vi "Extract RSSI Measurement from String.vi"(11 "Normal Event Log String":string="LogNum=1\r\nCount=7\r\nSerial=0\r\n\r\nTimestamp=4472778\r\nEvent=2308\r\nDescription= E_LOG_MICS_RSSI\r\nEventData[0]=1E\r\nEventData[1]=00\r\nEventData[2]=00\r\nEventData[3]=00\r\n\r\nTimestamp=4472802\r\nEvent=2308\r\nDescription= E_LOG_MICS_RSSI\r\nEventData[0]=0B\r\nEventData[1]=00\r\nEventData[2]=00\r\nEventData[3]=00\r\n\r\nTimestamp=4472828\r\nEvent=2308\r\nDescription= E_LOG_MICS_RSSI\r\nEventData[0]=00\r\nEventData[1]=00\r\nEventData[2]=00\r\nEventData[3]=00\r\n\r\nTimestamp=4472854\r\nEvent=2308\r\nDescription= E_LOG_MICS_RSSI\r\nEventData[0]=00\r\nEventData[1]=00\r\nEventData[2]=00\r\nEventData[3]=00\r\n\r\nTimestamp=4475025\r\nEvent=2121\r\nDescription= Event log was read\r\nEventData[0]=00\r\nEventData[1]=00\r\nEventData[2]=00\r\nEventData[3]=00\r\n\r\nTimestamp=9513895\r\nEvent=2121\r\nDescription= Event log was read\r\nEventData[0]=00\r\nEventData[1]=00\r\nEventData[2]=00\r\nEventData[3]=00\r\n\r\nTimestamp=9578215\r\nEvent=2121\r\nDescription= Event log was read\r\nEventData[0]=00\r\nEventData[1]=00\r\nEventData[2]=00\r\nEventData[3]=00") -> (2 "RSSI Values":u32[](array[numeric]), 3 "RSSI Values (String, HEX)":string[](array[string]))   [LabVIEW 2010]
doc: "This function converts a string containg the IPG VBAT ADC count into volts.\n\nThe IPG VBAT ADC is 12-bit unsigned, full scale is 5.00 volts.\nThe ADC scale factor is 0.001221001 per ADC bit. (4095 * 0.001221001 = 5.0000 volts)"
panel:
  out "tokens":string[](array[string])
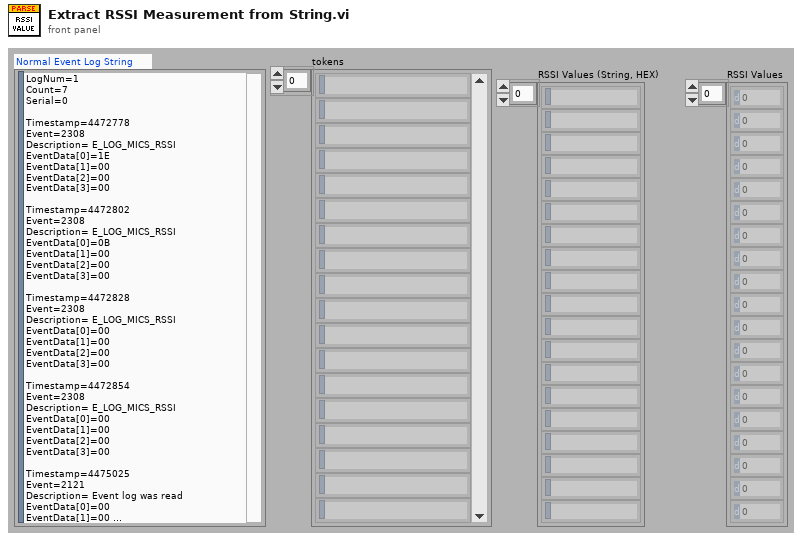
[diagram p1: front panel]
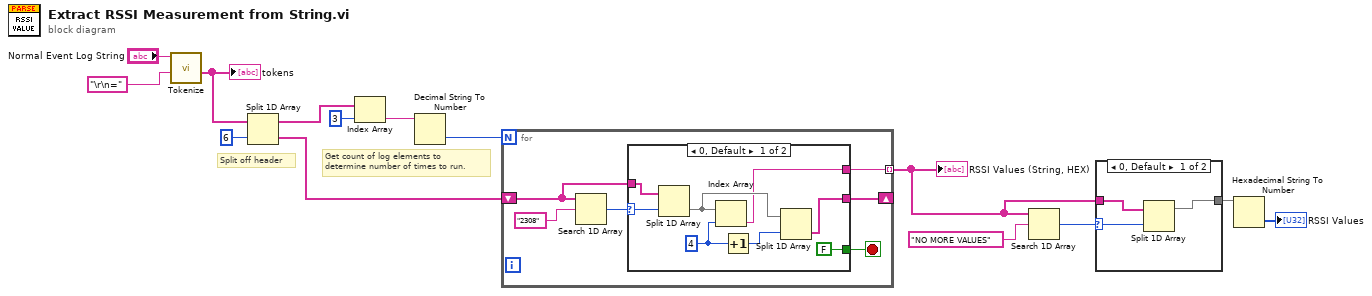
[diagram p0: block diagram]
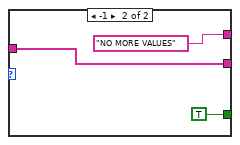
[diagram p3: hidden frame]
diagram:
  # "Get count of log elements to\ndetermine number of times to run."
  # "Split off header"
  n1 = call "Tokenize.vi"("delimiters (\\s,\\t,\\r,\\n,=)"="\r\n=" ("delimiters (\\s,\\t,\\r,\\n,=)"), "input string"="Normal Event Log String") -> ("tokens"=w12:string[])  [unwired: 3 in, 2 out]
  "tokens" <- w12
  n2 = Split 1D Array(array=w12, index=6) -> (first subarray=w10:string[], second subarray=w11:string[])
  n3 = Index Array(array=w10, index=3) -> (element=w8:string)
  n4 = Decimal String To Number(string=w8) -> (number=w7:i32)  [unwired: 2 in, 1 out]
  n5 = for {
    N: w7 -> [_]
    shift-right: [w18] -> _
    shift-left: w11 -> [w19]
    tunnel: [w17] -> w3 mode=indexing
    stop <- w15 stop-if-true
    n6 = Search 1D Array(1D array=w19, element="2308") -> (index of element=w16:i32)  [unwired: 1 in]
    n7 = case shown="0, Default" w16 {
      selector: w16 -> [w22 _]
      tunnel: w19 -> [w28 w30]
      tunnel: [w24 w30] -> w18
      tunnel: [w23 "NO MORE VALUES" ("token string")] -> w17
      tunnel: [FALSE TRUE] -> w15
      frame 0, Default {
        w25 = 4 ("y")
        n8 = Split 1D Array(array=w28, index=w22) -> (second subarray=w27:string[])  [unwired: 1 out]
        n9 = Index Array(array=w27, index=w25) -> (element=w23:string)
        n10 = Increment(x=w25) -> (x+1=w26:i32)
        n11 = Split 1D Array(array=w27, index=w26) -> (second subarray=w24:string[])  [unwired: 1 out]
      }
      frame -1 {
      }
    }
  }
  "RSSI Values (String, HEX)" <- w3
  n12 = Search 1D Array(1D array=w3, element="NO MORE VALUES" ("token string")) -> (index of element=w4:i32)  [unwired: 1 in]
  n13 = case shown="0, Default" w4 {
    selector: w4 -> [w34 _]
    tunnel: [w32 w35] -> w2
    tunnel: w3 -> [w33 w35]
    frame 0, Default {
      n14 = Split 1D Array(array=w33, index=w34) -> (first subarray=w32:string[])  [unwired: 1 out]
    }
    frame -1 {
    }
  }
  n15 = Hexadecimal String To Number(string=w2) -> (number=→"RSSI Values":u32[])  [unwired: 2 in, 1 out]
